vi "CMN_SetMaxElePerBuffer.vi"(10 "maxele_per_read_buffer":i32=65536, 11 "Database RefNum":T1) -> ()   [LabVIEW 2016]
uses:
  DBSHAND/private/vis/DatabaseHand_RefNum.ctl
  DBSHAND/private/vis/DatabaseHand_Element_Set(I32).vi
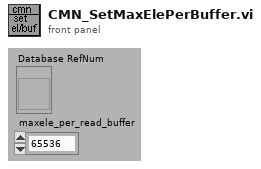
[diagram p1: front panel]
types:
  T1 = typedef "DatabaseHand_RefNum.ctl" = refnum<vi>
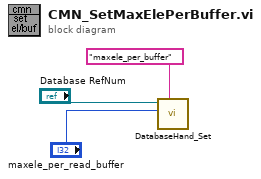
[diagram p0: block diagram]
diagram:
  n1 = call-poly "DatabaseHand_Set.vi"("name"="maxele_per_buffer", "value"="maxele_per_read_buffer", "Database RefNum in"="Database RefNum") -> ()  [unwired: 5 in, 4 out]
